vi "Mode 3 Process TRM File.vi"(8 "error in (no error)":errorcluster, 11 "Upload TR Module file":path) -> (0 "error out":errorcluster, 2 "Mode 3 Steps":T1[](array[typedef]), 3 "No file = True":bool)   [LabVIEW 2018]
uses:
  APARMainSubvis/UI temporary dialogs and VIs/Mode3FileRowData.ctl
  <vilib>/Utility/file.llb/Read Delimited Spreadsheet (string).vi
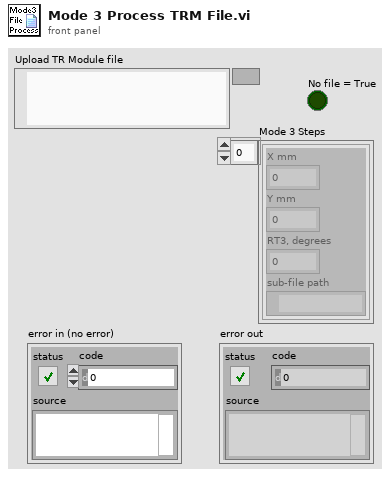
[diagram p1: front panel]
types:
  T1 = typedef "Mode3FileRowData.ctl" = cluster{"X mm":dbl, "Y mm":dbl, "RT3, degrees":dbl, "sub-file path":path}
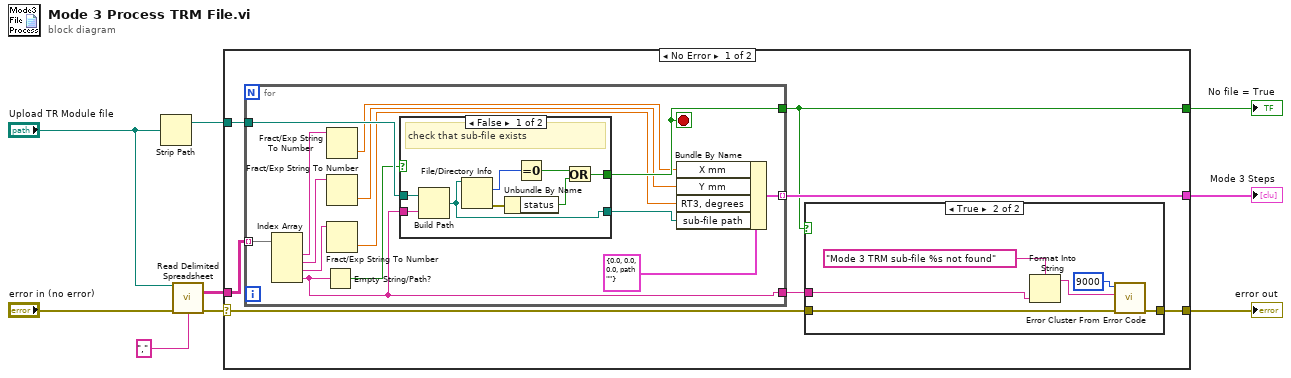
[diagram p0: block diagram]
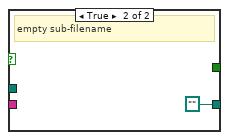
[diagram p3: hidden frame]
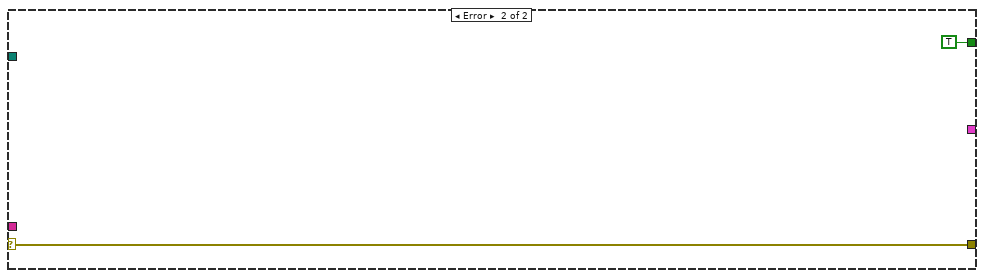
[diagram p4: hidden frame]
diagram:
  n1 = Strip Path(path="Upload TR Module file") -> (stripped path=w7:path)  [unwired: 1 out]
  n2 = call-poly <vilib>:"Read Delimited Spreadsheet.vi"("file path (dialog if empty)"="Upload TR Module file", "error in (no error)"="error in (no error)", "delimiter (\\t)"="," ("delimiter (\\t)")) -> ("all rows"=w8:string[][], "error out"=w3:errorcluster)  [unwired: 7 in, 4 out]
  n3 = case shown="No Error" w3 {
    selector: w3 -> [w13 w48]
    tunnel: w8 -> [w16 _]
    tunnel: w7 -> [w15 _]
    tunnel: [w11 TRUE] -> w5
    tunnel: [w14 _] -> w4
    tunnel: [w12 w48] -> w1
    frame No Error {
      n4 = for {
        tunnel: w16 -> [w37] mode=indexing
        tunnel: w15 -> [w34]
        tunnel: [w33] -> w11
        tunnel: [w30] -> w14 mode=indexing
        tunnel: [w27] -> w10
        stop <- w33 stop-if-true
        n5 = Index Array(array=w37) -> (element #1=w36:string, element #2=w35:string, element #3=w25:string, element #4=w27:string)  [unwired: 4 in]
        n6 = Empty String/Path?(string/path=w27) -> (empty?=w29:bool)
        n7 = Fract/Exp String To Number(string=w36) -> (number=w32:dbl)  [unwired: 3 in, 1 out]
        n8 = Fract/Exp String To Number(string=w35) -> (number=w31:dbl)  [unwired: 3 in, 1 out]
        n9 = Fract/Exp String To Number(string=w25) -> (number=w24:dbl)  [unwired: 3 in, 1 out]
        n10 = case shown="False" w29 {
          tunnel: w34 -> [w45 _]
          tunnel: [w40 _] -> w33
          tunnel: [w39 path ""] -> w26
          tunnel: w27 -> [w38 _]
          frame False {
            # "check that sub-file exists"
            n11 = Build Path(base path=w45, name or relative path=w38) -> (appended path=w39:path)
            n12 = File/Directory Info(path=w39) -> (size=w42:i64, error out=w41:errorcluster)  [unwired: 1 in, 5 out]
            n13 = Unbundle By Name(w41) -> ("status"=w43:bool)
            n14 = Equal To 0?(x=w42) -> (x = 0?=w44:bool)
            n15 = Or(x=w44, y=w43) -> (x .or. y?=w40:bool)
          }
          frame True {
            # "empty sub-filename"
          }
        }
        n16 = Bundle By Name(cluster=T1 {"X mm"=0.0, "Y mm"=0.0, "RT3, degrees"=0.0, "sub-file path"=path ""} ("Cluster"), "X mm"=w32, "Y mm"=w31, "RT3, degrees"=w24, "sub-file path"=w26) -> (w30:T1)
      }
      n17 = case shown="True" w11 {
        tunnel: w13 -> [w17 w23]
        tunnel: [w17 w22] -> w12
        tunnel: w10 -> [_ w21]
        frame False {
        }
        frame True {
          n18 = Format Into String(format string="Mode 3 TRM sub-file %s not found", w21) -> (resulting string=w19:string)  [unwired: 2 in, 1 out]
          n19 = call <vilib>:"Error Cluster From Error Code.vi"("error in (no error)"=w23, "error message (\"\")"=w19, "error code (0)"=9000) -> ("error out"=w22:errorcluster)  [unwired: 6 in]
        }
      }
    }
    frame Error {
    }
  }
  "No file = True" <- w5
  "Mode 3 Steps" <- w4
  "error out" <- w1
